vi "getPacketFromRecord.vi"(0 "foundPack":u8[][](array[numeric]) format="%02x") -> (4 "PacketArray":T1[](array[typedef]))   [LabVIEW 2023]
uses:
  controls/glbRoboterData.ctl
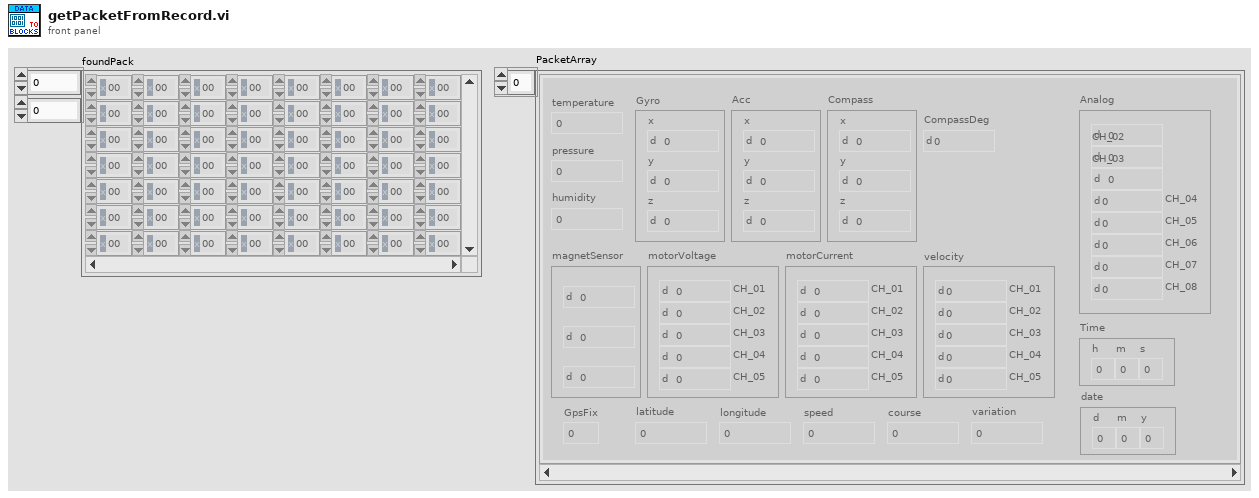
[diagram p1: front panel]
types:
  T1 = typedef "glbRoboterData.ctl" = cluster{"temperature":i16, "pressure":i16, "humidity":i16, "Gyro":cluster{"x":i16, "y":i16, "z":i16}, "Acc":cluster{"x":i16, "y":i16, "z":i16}, "Compass":cluster{"x":i16, "y":i16, "z":i16}, "CompassDeg":u32, "Analog":cluster{"CH_01":i16, "CH_02":i16, "CH_03":i16, "CH_04":i16, "CH_05":i16, "CH_06":i16, "CH_07":i16, "CH_08":i16}, "magnetSensor":cluster{"x":i16, "y":i16, "z":i16}, "motorVoltage":cluster{"CH_01":i16, "CH_02":i16, "CH_03":i16, "CH_04":i16, "CH_05":i16}, "motorCurrent":cluster{"CH_01":i16, "CH_02":i16, "CH_03":i16, "CH_04":i16, "CH_05":i16}, "velocity":cluster{"CH_01":i16, "CH_02":i16, "CH_03":i16, "CH_04":i16, "CH_05":i16}, "GpsFix":u8, "latitude":sgl, "longitude":sgl, "speed":sgl, "course":sgl, "variation":sgl, "Time":cluster{"h":u8, "m":u8, "s":u8}, "date":cluster{"d":u8, "m":u8, "y":u8}}
  T2 = enum16{"big-endian, network order", "native, host order", "little-endian"}
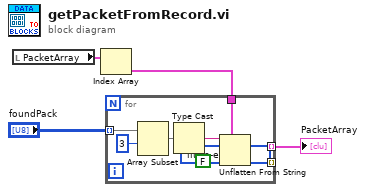
[diagram p0: block diagram]
diagram:
  n1 = local read "PacketArray"() -> (w2:T1[])
  n2 = Index Array(array=w2) -> (element=w1:T1)  [unwired: 1 in]
  n3 = for {
    tunnel: "foundPack" -> [w13] mode=indexing
    tunnel: [w10] -> w3 mode=indexing
    tunnel: w1 -> [w11]
    tunnel: [w9] -> _ mode=indexing
    n4 = Array Subset(array=w13, index=3) -> (w8:u8[])  [unwired: 1 in]
    n5 = Type Cast(x=w8) -> (*(type *) &x=w7:string)  [unwired: 1 in]
    n6 = Unflatten From String(type=w11, binary string=w7, data includes array or string size? (T)=FALSE, byte order (0:big-endian, network order)=T2."little-endian") -> (value=w10:T1, error out=w9:errorcluster)  [unwired: 1 in, 1 out]
  }
  "PacketArray" <- w3
